vi "Read Module Reporting.vi"(7 "Module ID":string, 8 "error in":errorcluster, 11 "Standard Engine Repo Data in":refnum<class "Standard Engine Configuration.lvclass">) -> (0 "error out":errorcluster, 2 "error tag":string, 3 "Standard Engine Repo Data out":refnum<class "Standard Engine Configuration.lvclass">)   [LabVIEW 2013, in "Standard Engine Configuration.lvclass"]
uses:
  Standard Engine Configuration.lvclass
  Standard Engine Configuration.lvclass/Standard Engine Configuration.ctl
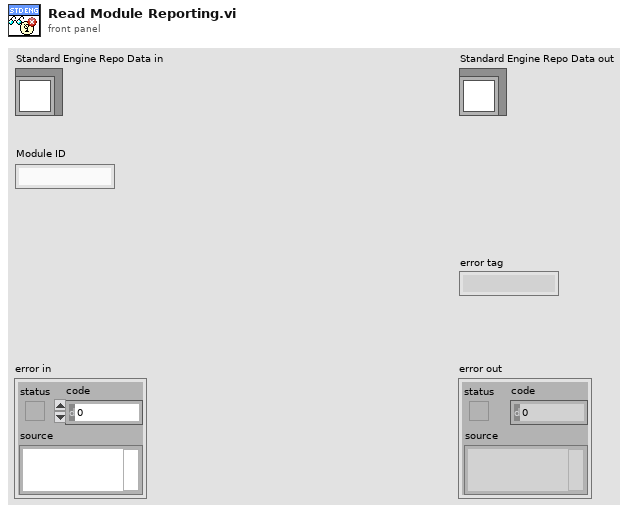
[diagram p1: front panel]
types:
  T1 = typedef "Standard Engine Configuration.lvclass/Module Specific Configuration.ctl" = cluster{"Module ID":string, "Module Decimation":T2, "Module Error Configuration":T3, "execution order priority":i32, "async?":bool, "error tag":string}
  T2 = typedef "Standard Engine Configuration.lvclass/Module Decimation.ctl" = cluster{"Decimation":u16, "Offset":u16}
  T3 = typedef "Standard Engine Configuration.lvclass/Module Error Configuration.ctl" = cluster{"Module Error Configuration":T4[]}
  T4 = typedef "Standard Engine Configuration.lvclass/Error Actions By Category.ctl" = cluster{"error classification":T5, "Error Actions":T6[]}
  T5 = typedef "TBM module execution interface.lvclass/error classification.ctl" = enum16{"unknown", "none", "trivial", "recoverable", "critical"}
  T6 = typedef "Standard Engine Configuration.lvclass/Error Actions.ctl" = enum16{"Clear", "Notify", "Stop Component", "Stop Engine", "Safe State", "Attempt Recovery"}
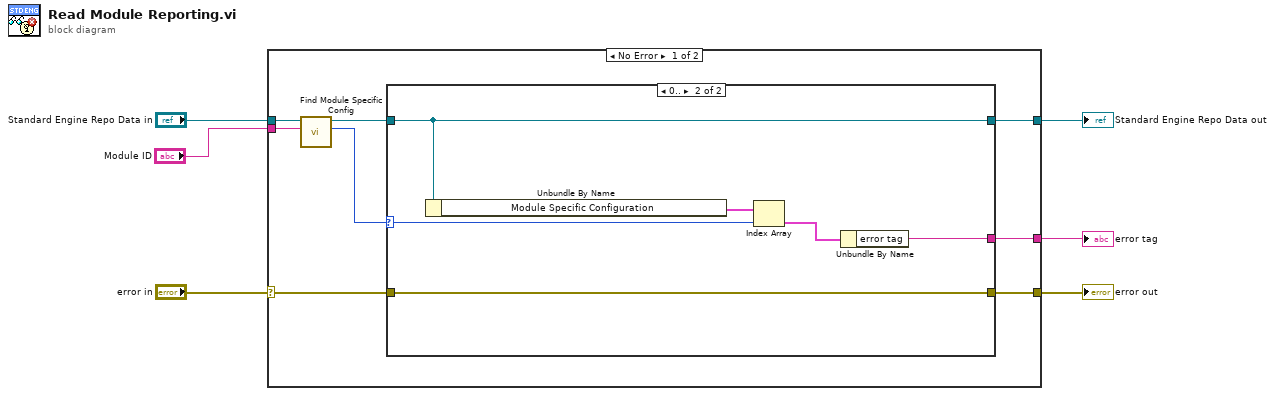
[diagram p0: block diagram]
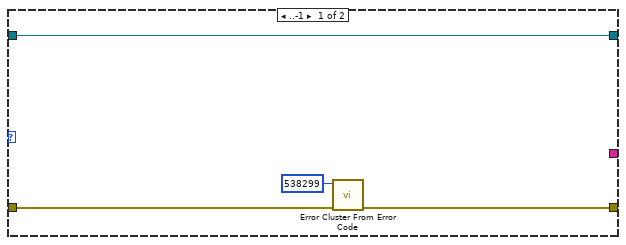
[diagram p2: hidden frame]
diagram:
  n1 = case shown="No Error" "error in" {
    selector: "error in" -> [w10 w26]
    tunnel: "Standard Engine Repo Data in" -> [w14 w25]
    tunnel: "Module ID" -> [w13 _]
    tunnel: [w8 w25] -> w2
    tunnel: [w9 w26] -> w4
    tunnel: [w7 _] -> w1
    frame No Error {
      n2 = call "Find Module Specific Config.vi"("Module ID"=w13, "Standard Engine Repo Data in"=w14) -> ("Index"=w11:i32, "Standard Engine Repo Data out"=w12:refnum<class "Standard Engine Configuration.lvclass">)  [unwired: 8 in]
      n3 = case shown="0.." w11 {
        selector: w11 -> [_ w21]
        tunnel: w12 -> [w18 w22]
        tunnel: w10 -> [w17 w20]
        tunnel: [w16 w20] -> w9
        tunnel: [w18 w22] -> w8
        tunnel: [_ w19] -> w7
        frame ..-1 {
          n4 = call <vilib>:"Error Cluster From Error Code.vi"("error in (no error)"=w17, "error code (0)"=538299) -> ("error out"=w16:errorcluster)  [unwired: 7 in]
        }
        frame 0.. {
          n5 = Unbundle By Name(w22) -> ("Module Specific Configuration"=w24:T1[])
          n6 = Index Array(array=w24, index=w21) -> (element=w23:T1)
          n7 = Unbundle By Name(w23) -> ("error tag"=w19:string)
        }
      }
    }
    frame Error {
    }
  }
  "error out" <- w4
  "Standard Engine Repo Data out" <- w2
  "error tag" <- w1
